vi "Create synth image from array.vi"() -> ()   [LabVIEW 2015]
panel:
  out "Array 2":u16[](array[numeric])
  in  "File Path":path
  out "Image Out":T1(plugin-control)
  in  "Array":bool[][](array[boolean])=[[FALSE, FALSE, FALSE, FALSE, FALSE, FALSE, FALSE, FALSE, FALSE, FALSE], [FALSE, FALSE, FALSE, FALSE, FALSE, FALSE, FALSE, FALSE, FALSE, FALSE], [FALSE, FALSE, FALSE, FALSE, FALSE, FALSE, FALSE, FALSE, FALSE, FALSE], [FALSE, FALSE, FALSE, FALSE, FALSE, FALSE, FALSE, FALSE, FALSE, FALSE], [FALSE, FALSE, FALSE, FALSE, FALSE, FALSE, FALSE, FALSE, FALSE, FALSE], [FALSE, FALSE, FALSE, FALSE, FALSE, FALSE, FALSE, FALSE, FALSE, FALSE], [FALSE, FALSE, FALSE, FALSE, FALSE, FALSE, FALSE, FALSE, FALSE, FALSE], [FALSE, FALSE, FALSE, FALSE, FALSE, FALSE, FALSE, FALSE, FALSE, FALSE], [FALSE, FALSE, FALSE, FALSE, FALSE, FALSE, FALSE, FALSE, FALSE, FALSE], [FALSE, FALSE, FALSE, FALSE, FALSE, FALSE, FALSE, FALSE, FALSE, FALSE]]
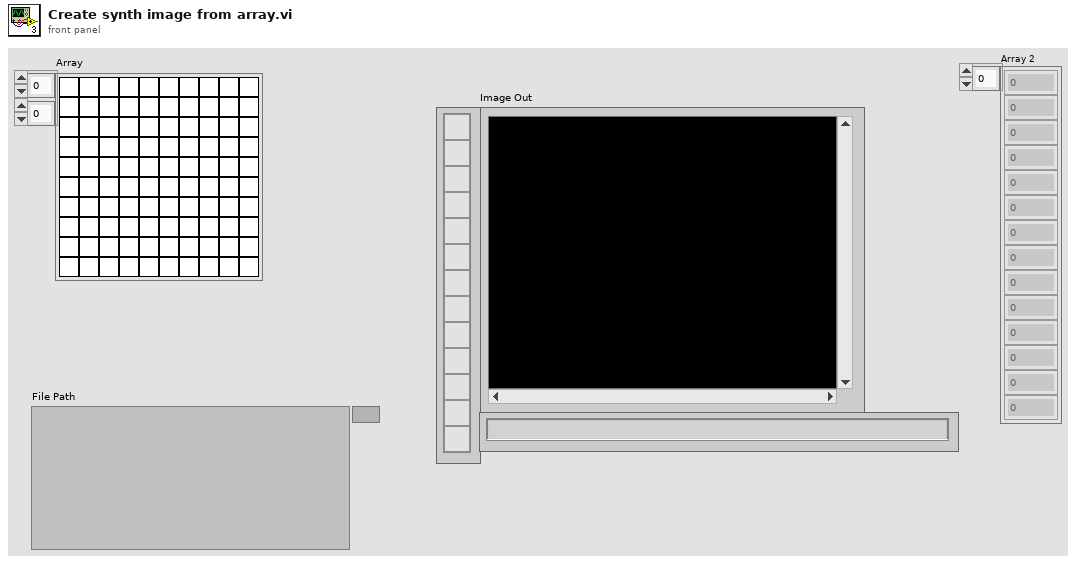
[diagram p1: front panel]
types:
  T1 = typedef "IMAQ Image.ctl" = refnum<image>
  T2 = typedef "Image Type" = u32
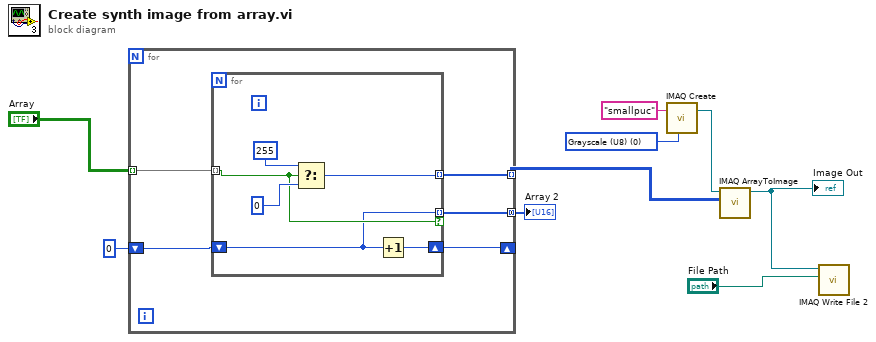
[diagram p0: block diagram]
diagram:
  w5 = T2 0 items=["Grayscale (U8)", "Grayscale (I16)", "Grayscale (SGL)", "Complex (CSG)", "RGB (U32)", "HSL (U32)", "RGB (U64)", "Grayscale (U16)"] ("Image Type")
  n1 = for {
    tunnel: "Array" -> [w14] mode=indexing
    tunnel: [w13] -> w8 mode=indexing
    shift-right: [w11] -> _
    shift-left: u16 0 -> [w12]
    tunnel: [w10] -> w1 mode=concatenating
    n2 = for {
      tunnel: w14 -> [w16] mode=indexing
      tunnel: [w18] -> w13 mode=indexing
      shift-right: [w17] -> w11
      shift-left: w12 -> [w15]
      tunnel: [w15] -> w10 mode=indexing if=w16
      n3 = Select(t=u8 255, s=w16, f=u8 0) -> (s? t:f=w18:u8)
      n4 = Increment(x=w15) -> (x+1=w17:u16)
    }
  }
  "Array 2" <- w1
  n5 = call "IMAQ Create"("Image Name"="smallpuc", "Image Type"=w5) -> ("New Image"=w6:T1)  [unwired: 3 in, 1 out]
  n6 = call "IMAQ ArrayToImage"("Image Pixels (U8)"=w8, "Image"=w6) -> ("Image Out"=w4:T1)  [unwired: 8 in, 1 out]
  "Image Out" <- w4
  n7 = call-poly "IMAQ Write File 2"("File Path"="File Path", "Image"=w4) -> ()  [unwired: 8 in, 2 out]
